vi "3.2.vi"() -> ()   [LabVIEW 2017]
panel:
  out "数值 3":dbl
  in  "数值 2":dbl
  in  "数值":dbl
  in  "枚举":enum16{"相除", "相乘", "相减", "相加"}(ring)
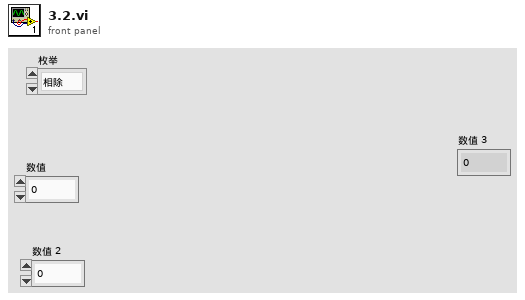
[diagram p1: front panel]
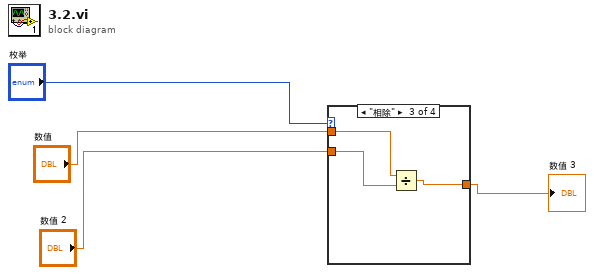
[diagram p0: block diagram]
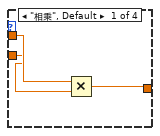
[diagram p2: hidden frame]
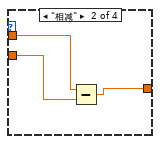
[diagram p3: hidden frame]
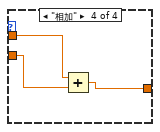
[diagram p4: hidden frame]
diagram:
  n1 = case shown="\"相除\"" "枚举" {
    tunnel: "数值" -> [w7 w10 w12 w15]
    tunnel: "数值 2" -> [w6 w9 w11 w14]
    tunnel: [w5 w8 w13 w16] -> w3
    frame "相乘", Default {
      n2 = Multiply(x=w7, y=w6) -> (x*y=w5:dbl)
    }
    frame "相减" {
      n3 = Subtract(x=w10, y=w9) -> (x-y=w8:dbl)
    }
    frame "相除" {
      n4 = Divide(x=w12, y=w11) -> (x/y=w13:dbl)
    }
    frame "相加" {
      n5 = Add(x=w15, y=w14) -> (x+y=w16:dbl)
    }
  }
  "数值 3" <- w3
